vi "Get Command Parameters.vi"(8 "error in (no error)":errorcluster, 10 "Command Parameters In":T1 {"Linkages"."Channel Ref" format="%.0x"}, 11 "Item Ref in":T4 format="%.0x") -> (0 "error out":errorcluster, 2 "Command Parameters Out":T1 {"Linkages"."Channel Ref" format="%.0x"}, 3 "Item Ref out":T4 format="%.0x")   [LabVIEW 2018, in "Instrument Addon Scripting API.lvlib"]
uses:
  Instrument Addon Scripting API.lvlib
  <vilib>/NI Veristand/Custom Device API/Custom Device Item Ref.ctl
  TypeDefs/Command Settings.ctl
  TypeDefs/Padding.ctl
  TypeDefs/Linked Channel.ctl
  Addon/Addon Shared/SubVIs/Constants.vi
  <vilib>/NI Veristand/Custom Device API/Get Item Property (String).vi
  <vilib>/NI Veristand/Custom Device API/Get Item Property (String Array).vi
  <vilib>/NI Veristand/Custom Device API/Get Item Property (U32 Array).vi
  <vilib>/NI Veristand/Custom Device API/Get Item Property (Boolean).vi
  <vilib>/NI Veristand/Custom Device API/Get Item Property (U32).vi
  Addon/Addon Shared/Instrument Addon Shared.lvlib
  <vilib>/NI VeriStand/Custom Device API/Custom Device API.lvlib
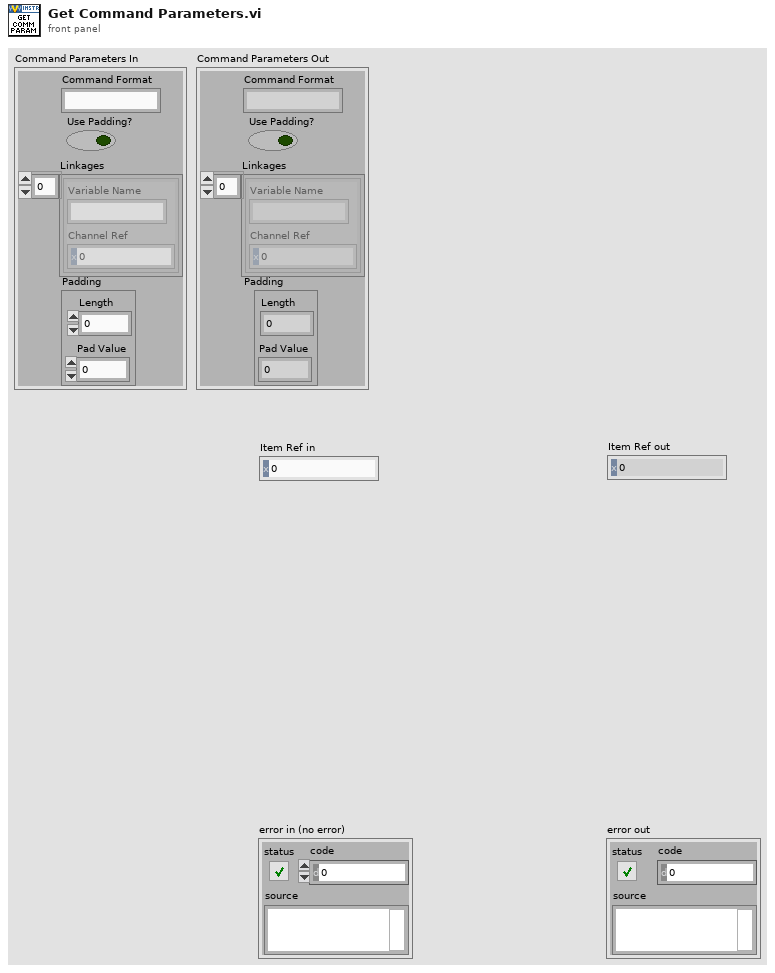
[diagram p1: front panel]
types:
  T1 = typedef "Instrument Addon Scripting API.lvlib/Command Settings.ctl" = cluster{"Command Format":string, "Use Padding?":bool, "Padding":T2, "Linkages":T3}
  T2 = typedef "Instrument Addon Scripting API.lvlib/Padding.ctl" = cluster{"Length":u32, "Pad Value":u8}
  T3 = typedef "Instrument Addon Scripting API.lvlib/Linked Channel.ctl" = cluster{"Channel Ref":T4, "Variable Name":string}[]
  T4 = typedef "Custom Device API.lvlib/Custom Device Item Ref.ctl" = u64
  T5 = cluster{"Channel Ref":T4, "Variable Name":string}
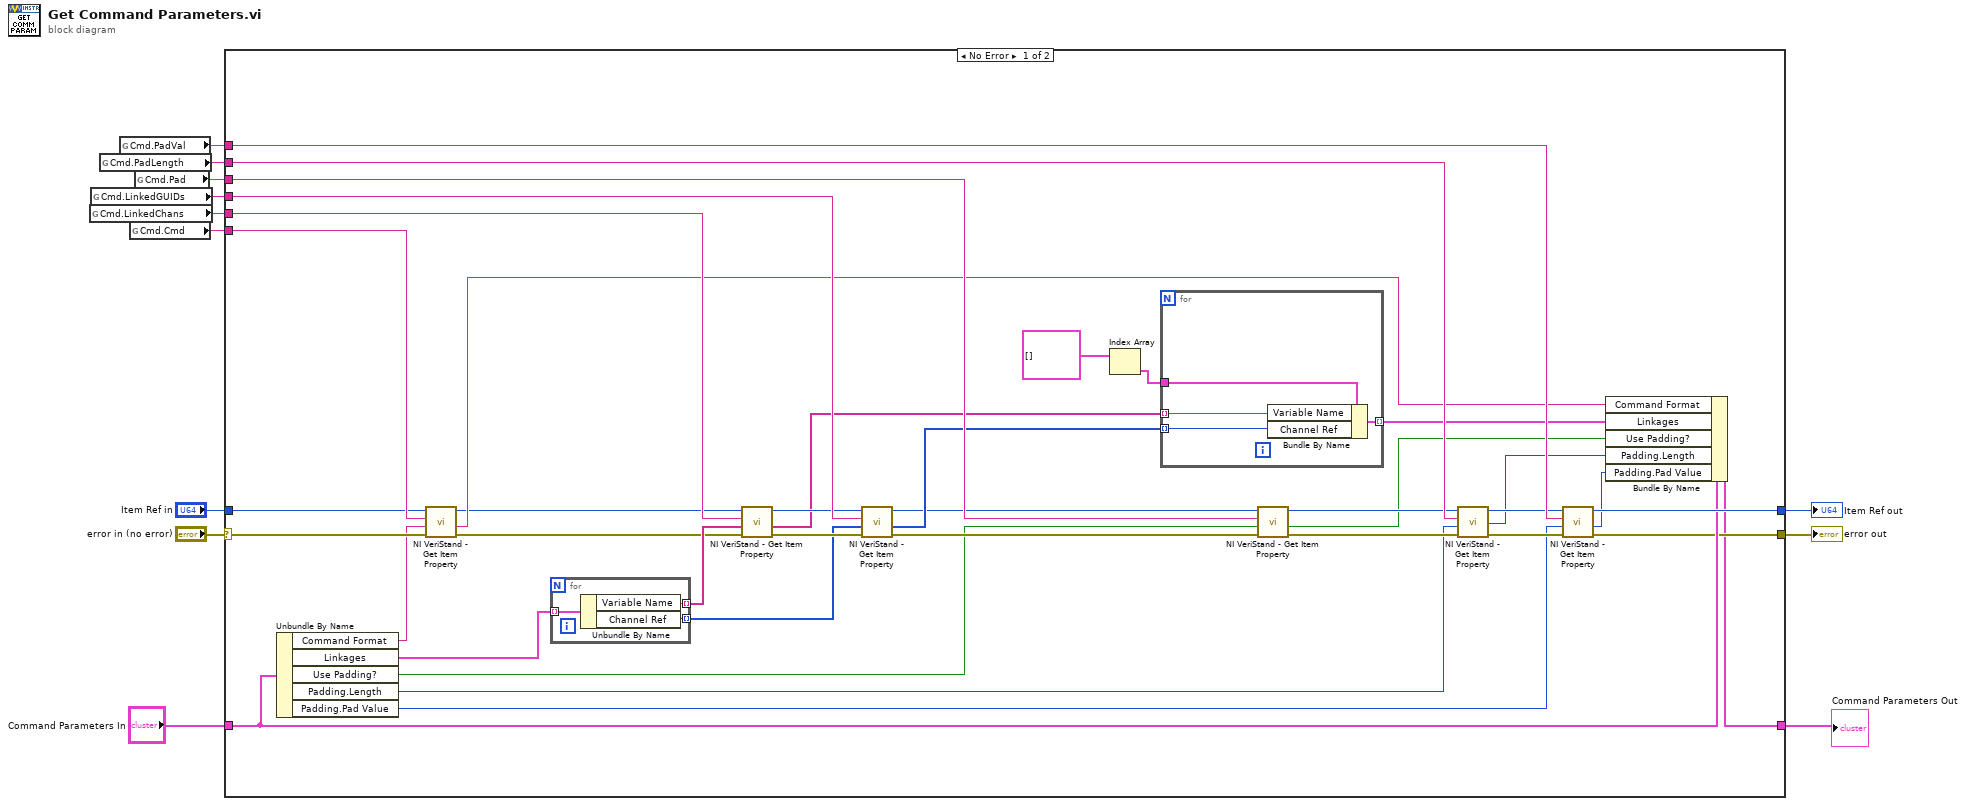
[diagram p0: block diagram]
diagram:
  n1 = global read "Constants.vi" "Cmd.LinkedChans"() -> (w6:string)
  n2 = global read "Constants.vi" "Cmd.LinkedGUIDs"() -> (w5:string)
  n3 = global read "Constants.vi" "Cmd.PadLength"() -> (w3:string)
  n4 = global read "Constants.vi" "Cmd.PadVal"() -> (w2:string)
  n5 = global read "Constants.vi" "Cmd.Cmd"() -> (w8:string)
  n6 = global read "Constants.vi" "Cmd.Pad"() -> (w4:string)
  n7 = case shown="No Error" "error in (no error)" {
    selector: "error in (no error)" -> [w45 w60]
    tunnel: w8 -> [w50 _]
    tunnel: [w49 w58] -> w11
    tunnel: "Item Ref in" -> [w48 w58]
    tunnel: "Command Parameters In" -> [w47 w59]
    tunnel: [w46 w60] -> w10
    tunnel: [w44 w59] -> w7
    tunnel: w6 -> [w43 _]
    tunnel: w5 -> [w42 _]
    tunnel: w4 -> [w41 _]
    tunnel: w3 -> [w40 _]
    tunnel: w2 -> [w39 _]
    frame No Error {
      n8 = Unbundle By Name(w47) -> ("Command Format"=w34:string, "Linkages"=w33:T3, "Use Padding?"=w27:bool, "Padding.Length"=w25:u32, "Padding.Pad Value"=w24:u8)
      n9 = call-poly <vilib>:"NI VeriStand - Get Item Property.vi"("error in (no error)"=w45, "Default Value"=w34, "Property Name"=w50, "Item Ref in"=w48) -> ("error out"=w16:errorcluster, "Value"=w17:string, "Item Ref out"=w15:T4)  [unwired: 4 in, 1 out]
      n10 = for {
        tunnel: w33 -> [w57] mode=indexing
        tunnel: [w56] -> w32 mode=indexing
        tunnel: [w55] -> w31 mode=indexing
        n11 = Unbundle By Name(w57) -> ("Variable Name"=w56:string, "Channel Ref"=w55:T4)
      }
      n12 = call-poly <vilib>:"NI VeriStand - Get Item Property.vi"("error in (no error)"=w16, "Default Value"=w32, "Property Name"=w43, "Item Ref in"=w15) -> ("error out"=w38:errorcluster, "Value"=w28:string[], "Item Ref out"=w30:T4)  [unwired: 4 in, 1 out]
      n13 = call-poly <vilib>:"NI VeriStand - Get Item Property.vi"("error in (no error)"=w38, "Default Value"=w31, "Property Name"=w42, "Item Ref in"=w30) -> ("error out"=w37:errorcluster, "Value"=w29:u32[], "Item Ref out"=w26:T4)  [unwired: 4 in, 1 out]
      n14 = Index Array(array=T3 [] ("Linkages")) -> (element=w13:T5)  [unwired: 1 in]
      n15 = for {
        tunnel: w29 -> [w53] mode=indexing
        tunnel: w28 -> [w52] mode=indexing
        tunnel: [w54] -> w21 mode=indexing
        tunnel: w13 -> [w51]
        n16 = Bundle By Name(cluster=w51, "Variable Name"=w52, "Channel Ref"=w53) -> (w54:T5)
      }
      n17 = call-poly <vilib>:"NI VeriStand - Get Item Property.vi"("error in (no error)"=w37, "Default Value"=w27, "Property Name"=w41, "Item Ref in"=w26) -> ("error out"=w36:errorcluster, "Value"=w20:bool, "Item Ref out"=w22:T4)  [unwired: 4 in, 1 out]
      n18 = call-poly <vilib>:"NI VeriStand - Get Item Property.vi"("error in (no error)"=w36, "Default Value"=w25, "Property Name"=w40, "Item Ref in"=w22) -> ("error out"=w35:errorcluster, "Value"=w19:u32, "Item Ref out"=w23:T4)  [unwired: 4 in, 1 out]
      n19 = call-poly <vilib>:"NI VeriStand - Get Item Property.vi"("error in (no error)"=w35, "Default Value"=w24, "Property Name"=w39, "Item Ref in"=w23) -> ("error out"=w46:errorcluster, "Value"=w18:u32, "Item Ref out"=w49:T4)  [unwired: 4 in, 1 out]
      n20 = Bundle By Name(cluster=w47, "Command Format"=w17, "Linkages"=w21, "Use Padding?"=w20, "Padding.Length"=w19, "Padding.Pad Value"=w18) -> (w44:T1)
    }
    frame Error {
    }
  }
  "error out" <- w10
  "Item Ref out" <- w11
  "Command Parameters Out" <- w7
